vi "GoTo PID rotação.vi"(8 "Position":dbl[](array[numeric]), 11 "Target":dbl[](array[numeric])) -> (3 "Velocity":dbl[](array[numeric]))   [LabVIEW 2016]
uses:
  <vilib>/Analysis/coordinate.llb/2D Cartesian Coordinate Rotation (Scalar).vi
  <vilib>/addons/control/pid/pid.llb/PID (DBL).vi
  <vilib>/addons/control/pid/NI_PID_pid.lvlib
  <vilib>/Analysis/NI_AALPro.lvlib
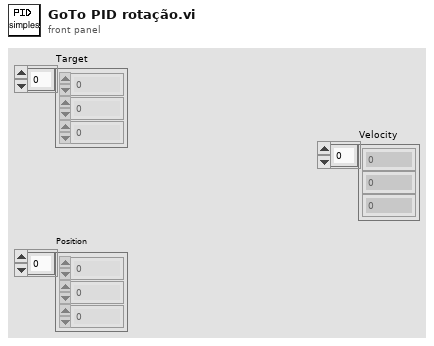
[diagram p1: front panel]
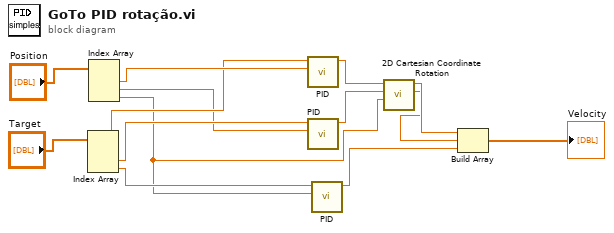
[diagram p0: block diagram]
diagram:
  n1 = Index Array(array="Target") -> (element #1=w10:dbl, element #2=w9:dbl, element #3=w7:dbl)  [unwired: 3 in]
  n2 = Index Array(array="Position") -> (element #1=w11:dbl, element #2=w8:dbl, element #3=w3:dbl)  [unwired: 3 in]
  n3 = call-poly <vilib>:"PID.vi"("process variable"=w11, "setpoint"=w10) -> ("output"=w5:dbl)  [unwired: 8 in, 1 out]
  n4 = call-poly <vilib>:"PID.vi"("process variable"=w8, "setpoint"=w9) -> ("output"=w4:dbl)  [unwired: 8 in, 1 out]
  n5 = call-poly <vilib>:"PID.vi"("process variable"=w3, "setpoint"=w7) -> ("output"=w6:dbl)  [unwired: 8 in, 1 out]
  n6 = call-poly <vilib>:"2D Cartesian Coordinate Rotation.vi"("theta"=w3, "y"=w4, "x"=w5) -> ("y out"=w1:dbl, "x out"=w2:dbl)  [unwired: 6 in, 1 out]
  n7 = Build Array(w2, w1, w6) -> (→"Velocity":dbl[])
